vi "DatabaseHand_GetSubElement.vi"(0 "Database RefNum in":T3, 7 "Object Data In":T2, 9 "Index":i32, 11 "error in (no error)":errorcluster) -> (4 "Database RefNum out":T3, 8 "Element found":T1, 15 "error out":errorcluster)   [LabVIEW 2016]
doc: "This VI finds the RefNum of an existing object with the input Name or creates a new object if the Name is not found or Name is unwired or an empty string.\nCopyright 2001 VI Engineering, Inc."
uses:
  DatabaseHand_RefNum.ctl
  DatabaseHand_Element.ctl
  DatabaseHan_DatabaseElement.ctl
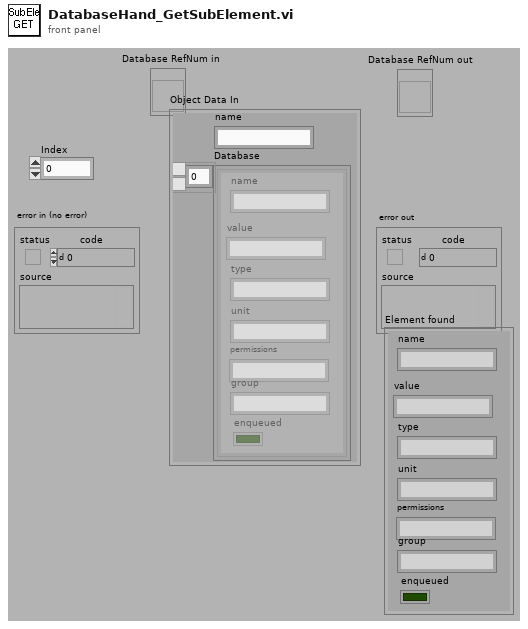
[diagram p1: front panel]
types:
  T1 = typedef "DatabaseHan_DatabaseElement.ctl" = cluster{"name":string, "value":string, "type":string, "unit":string, "permissions":string, "enqueued":bool, "group":string}
  T2 = typedef "DatabaseHand_Element.ctl" = cluster{"name":string, "Database":T1[]}
  T3 = typedef "DatabaseHand_RefNum.ctl" = refnum<vi>
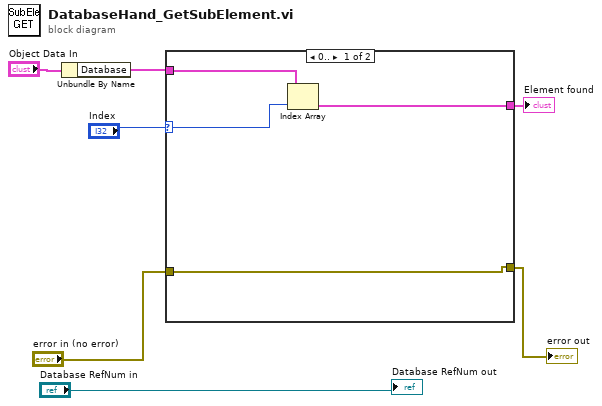
[diagram p0: block diagram]
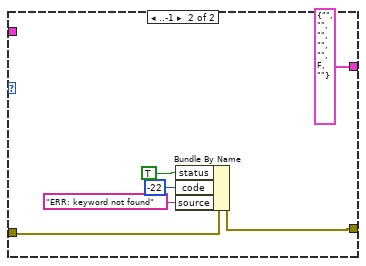
[diagram p2: hidden frame]
diagram:
  n1 = Unbundle By Name("Object Data In") -> ("Database"=w5:T1[])
  n2 = case shown="0.." "Index" {
    selector: "Index" -> [w10 _]
    tunnel: w5 -> [w11 _]
    tunnel: [w9 T1 {"name"="", "value"="", "type"="", "unit"="", "permissions"="", "enqueued"=FALSE, "group"=""} ("Object Data In")] -> w3
    tunnel: "error in (no error)" -> [w8 w16]
    tunnel: [w8 w15] -> w1
    frame 0.. {
      n3 = Index Array(array=w11, index=w10) -> (element=w9:T1)
    }
    frame ..-1 {
      n4 = Bundle By Name(cluster=w16, "status"=TRUE, "code"=-22, "source"="ERR: keyword not found") -> (w15:errorcluster)
    }
  }
  "error out" <- w1
  "Element found" <- w3
  "Database RefNum out" <- "Database RefNum in"
